vi "Transform.vi"(8 "error in (no error)":errorcluster caption="entrée d'erreur (pas d'erreur)", 9 "y":string[][](array[string]), 10 "X":string[][](array[string]), 11 "OrdinalEncoder.lvclass":refnum<class "OrdinalEncoder.lvclass">) -> (0 "error out":errorcluster caption="sortie d'erreur", 2 "Data":T1, 3 "OrdinalEncoder.lvclass":refnum<class "OrdinalEncoder.lvclass">)   [LabVIEW 2020, in "OrdinalEncoder.lvclass"]
doc: "Transform X to ordinal codes\n\nReturns : \n\n- X_out : sparse matrix or a 2-d array\nTransformed input."
uses:
  OrdinalEncoder.lvclass
  OrdinalEncoder.lvclass/OrdinalEncoder.ctl
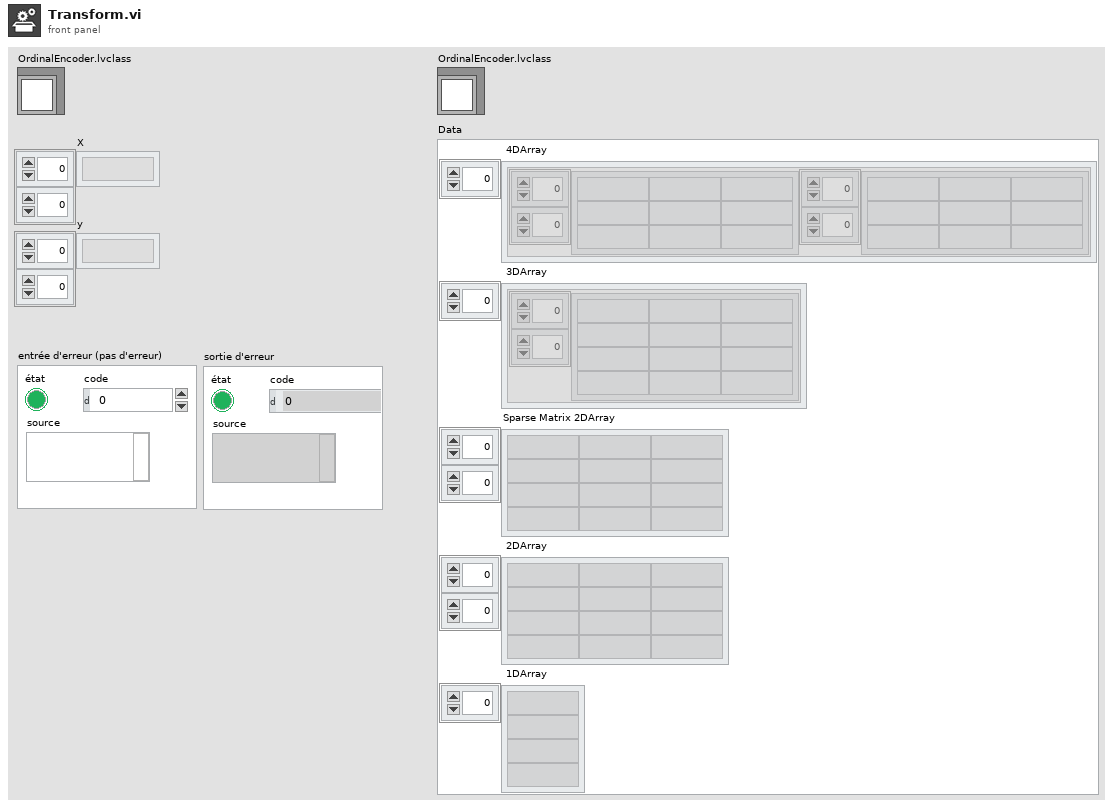
[diagram p1: front panel]
types:
  T1 = cluster{" 4DArray":cluster{"1":string[][], "2":string[][]}[], " 3DArray":cluster{"Tableau":string[][]}[], "Sparse Matrix 2DArray":string[][], " 2DArray":string[][], " 1DArray":string[]}
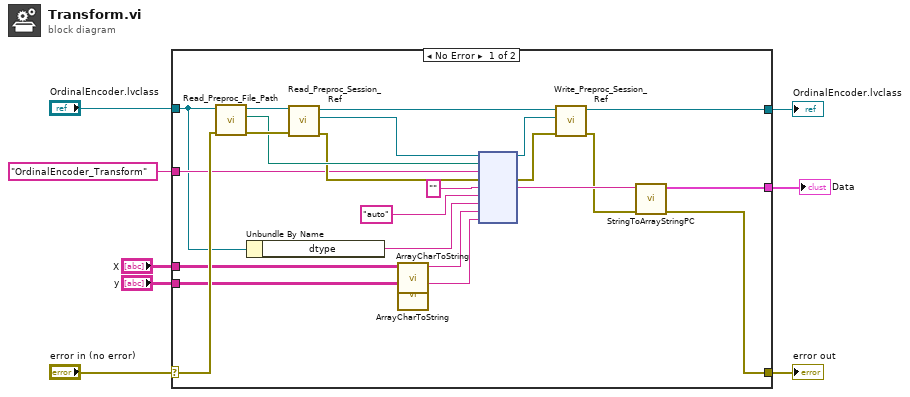
[diagram p0: block diagram]
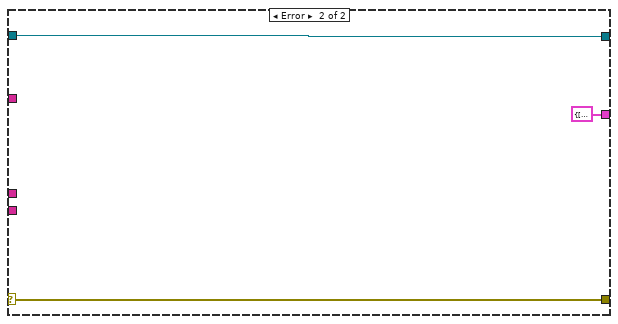
[diagram p2: hidden frame]
diagram:
  n1 = case shown="No Error" "error in (no error)" {
    selector: "error in (no error)" -> [w21 w34]
    tunnel: [w9 w34] -> w7
    tunnel: [w13 w33] -> w5
    tunnel: "OrdinalEncoder.lvclass" -> [w19 w33]
    tunnel: "OrdinalEncoder_Transform" ("Fonction") -> [w20 _]
    tunnel: [w10 T1 {" 4DArray"=[], " 3DArray"=[], "Sparse Matrix 2DArray"=[], " 2DArray"=[], " 1DArray"=[]} ("Data")] -> w3
    tunnel: "X" -> [w17 _]
    tunnel: "y" -> [w15 _]
    frame No Error {
      n2 = call-dynamic "Read_Preproc_File_Path.vi"("error in (no error)"=w21, "Python in"=w19) -> ("error out"=w30:errorcluster, "File_Path"=w27:path, "Python out"=w31:refnum<class "OrdinalEncoder.lvclass">)  [unwired: 7 in]
      n3 = Unbundle By Name(w19) -> ("dtype"=w22:string)
      n4 = call-dynamic "Read_Preproc_Session_Ref.vi"("error in (no error)"=w30, "Python in"=w31) -> ("error out"=w26:errorcluster, "Session_ref"=w28:refnum<k35>, "Python out"=w29:refnum<class "OrdinalEncoder.lvclass">)  [unwired: 7 in]
      n5 = call "ArrayCharToString.vi"("TAB"=w17) -> ("Instruction"=w16:string)  [unwired: 10 in]
      n6 = call "ArrayCharToString.vi"("TAB"=w15) -> ("Instruction"=w14:string)  [unwired: 10 in]
      n7 = node(w28, w27, w20, w26, "", "auto", w22, w16, w14) -> (w24:refnum<k35>, w25:errorcluster, w12:string)  [unwired: 4 in, 2 out]
      n8 = call-dynamic "Write_Preproc_Session_Ref.vi"("error in (no error)"=w25, "Session_ref"=w24, "Python in"=w29) -> ("error out"=w11:errorcluster, "Python out"=w13:refnum<class "OrdinalEncoder.lvclass">)  [unwired: 7 in]
      n9 = call "StringToArrayStringPC.vi"("sortie d'erreur"=w11, "Return value"=w12) -> ("sortie d'erreur"=w9:errorcluster, "Data"=w10:T1)  [unwired: 8 in]
    }
    frame Error {
    }
  }
  "error out" <- w7
  "OrdinalEncoder.lvclass" <- w5
  "Data" <- w3
